vi "Message Maker.vi"(7 "Message selector":T1=enum."2", 8 "error in (no error)":errorcluster, 9 "Numeric":dbl, 10 "String":string) -> (0 "error out":errorcluster, 2 "Message":string)   [LabVIEW 2019]
uses:
  controls/Message Selector.ctl
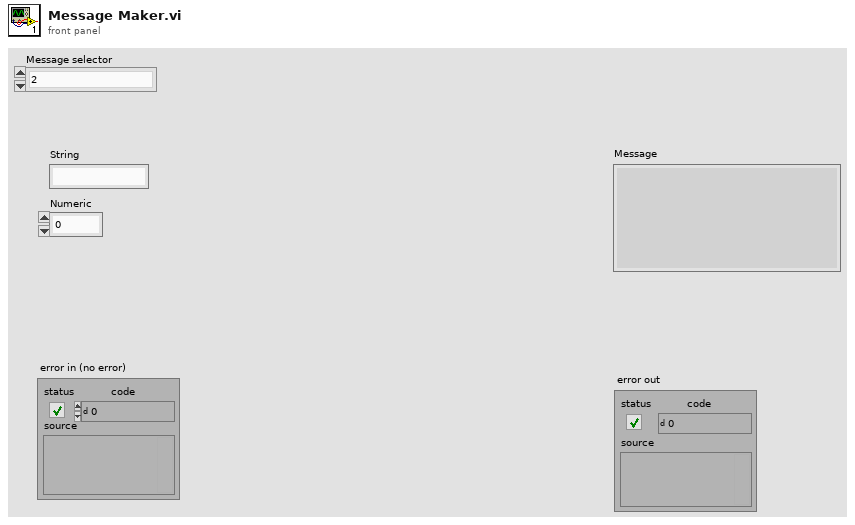
[diagram p1: front panel]
types:
  T1 = typedef "Message Selector.ctl" = enum16{"String 1", "DBL 2", "DBL 1", "1", "2"}
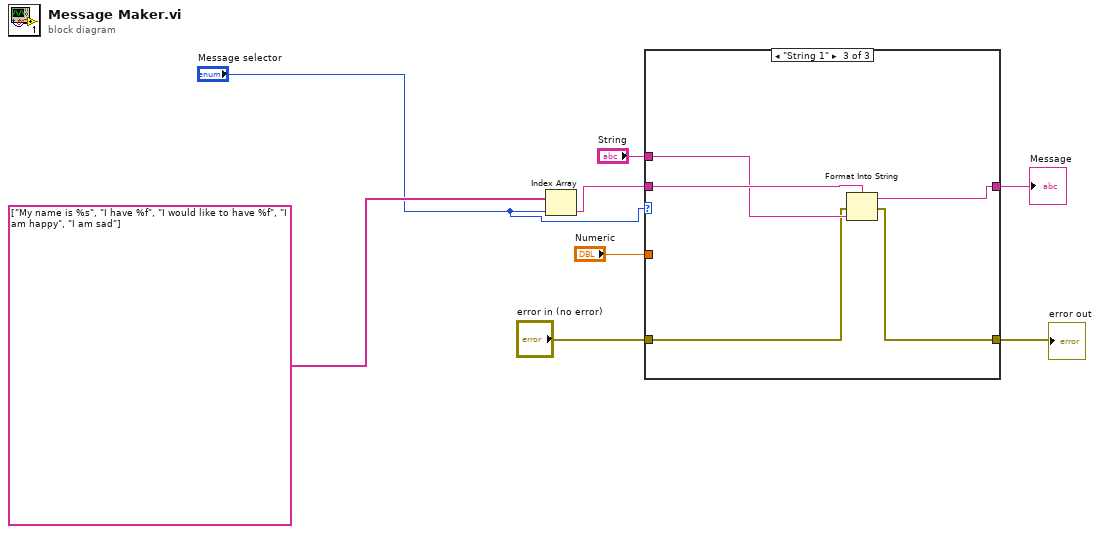
[diagram p0: block diagram]
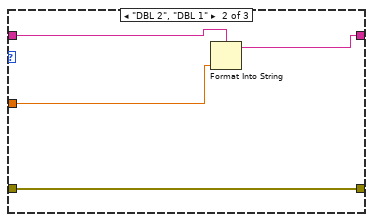
[diagram p3: hidden frame]
diagram:
  n1 = Index Array(array=string[] ["My name is %s", "I have %f", "I would like to have %f", "I am happy", "I am sad"], index="Message selector") -> (element=w4:string)
  n2 = case shown="\"String 1\"" "Message selector" {
    tunnel: "error in (no error)" -> [w9 w14 w16]
    tunnel: [w9 w14 w15] -> w6
    tunnel: w4 -> [w10 w13 w19]
    tunnel: [w10 w12 w18] -> w3
    tunnel: "Numeric" -> [_ w11 _]
    tunnel: "String" -> [_ _ w17]
    frame Default {
    }
    frame "DBL 2", "DBL 1" {
      n3 = Format Into String(format string=w13, w11) -> (resulting string=w12:string)  [unwired: 2 in, 1 out]
    }
    frame "String 1" {
      n4 = Format Into String(format string=w19, error in=w16, w17) -> (resulting string=w18:string, error out=w15:errorcluster)  [unwired: 1 in]
    }
  }
  "error out" <- w6
  "Message" <- w3
